vi "Valve-Close.vi"(7 "Device reference":refnum<vi>, 8 "error in (no error)":errorcluster, 9 "Eventstring":string="auto-generate") -> (0 "error out":errorcluster)   [LabVIEW 2015]
doc: "Closes a juicer valve.\n\nDevice reference: which valve?\nEventstring: used for timestamping\n--empty: no timestamp will be generated\n--unwired or \"auto-generate\": TS w/ default eventstring\n--otherwise: TS with user-provided string\n\nThe default eventstring is:\n[valve name].close\nwhere [valve name] is the referenced valve's front panel label text."
uses:
  Typedefs/Valve.ctl
  Rack/Typedefs/OutputRequest refnum.ctl
  Rack/Typedefs/OutputRequest.ctl
  Rack/Typedefs/InputData cluster.ctl
  Rack/Methods/Port drivers/DigitalInput-DataCluster.ctl
panel:
  # "(must be on same NI card)"
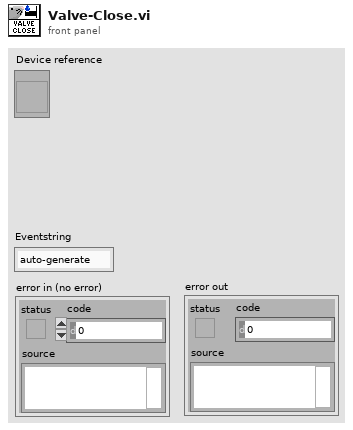
[diagram p1: front panel]
types:
  T1 = typedef "Valve.ctl" = cluster{"Settings":cluster{"Timestamp port name":string, "Port name":string, "Port index":i32}, "OutputRequest event ref":T2, "InputData reference":refnum<vi>, "Default length (ms)":i32}
  T2 = typedef "OutputRequest refnum.ctl" = refnum<user-event>
  T3 = typedef "OutputRequest.ctl" = cluster{"Target":string, "Command":string}
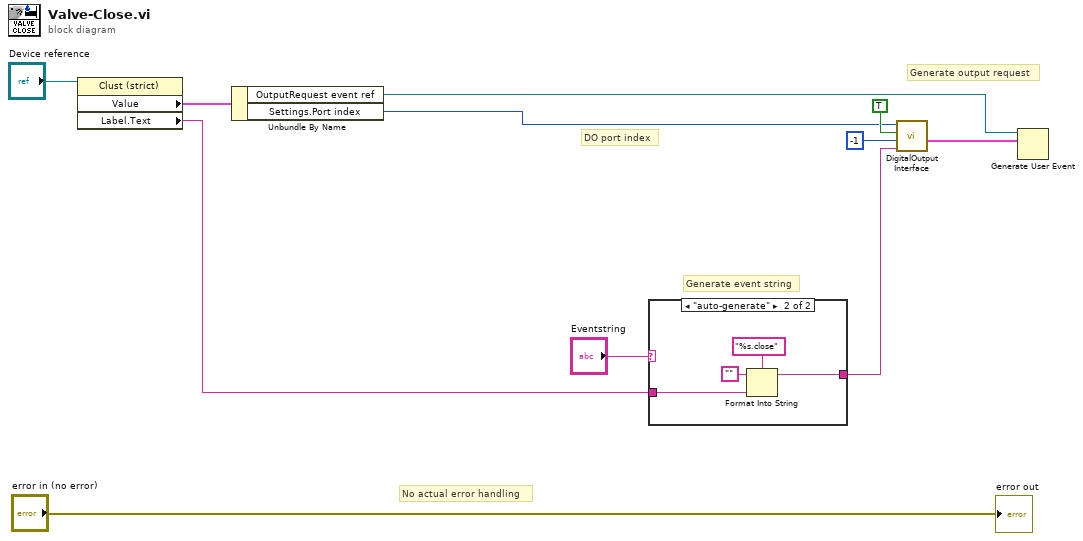
[diagram p0: block diagram]
diagram:
  # "No actual error handling"
  # "DO port index"
  # "Generate output request"
  # "Generate event string"
  n1 = property class="Clust (strict)"(reference="Device reference") -> ("Value"=w11:T1, "Label.Text"=w8:string)  [unwired: 1 in, 2 out]
  n2 = Unbundle By Name(w11) -> ("OutputRequest event ref"=w2:T2, "Settings.Port index"=w1:i32)
  n3 = case shown="\"auto-generate\"" "Eventstring" {
    selector: "Eventstring" -> [w12 _]
    tunnel: w8 -> [_ w14]
    tunnel: [w12 w13] -> w6
    frame Default {
      # "Use user-provided string"
    }
    frame "auto-generate" {
      n4 = Format Into String(format string="%s.close", initial string="", w14) -> (resulting string=w13:string)  [unwired: 1 in, 1 out]
    }
  }
  n5 = call "DigitalOutput Interface.vi"("Eventstring"=w6, "Pulse duration (-1 for cont.)"=-1, "On/off"=TRUE, "Port index"=w1) -> ("OutputRequest"=w5:T3)  [unwired: 7 in]
  n6 = Generate User Event(user event=w2, event data cluster=w5) -> ()  [unwired: 2 in, 2 out]
  "error out" <- "error in (no error)"
